vi "Adapt Cluster to Class.vi"() -> ()   [LabVIEW 2020]
doc: "This VI demonstrates a function of the GCraftsman JSON Serialization Toolkit.\n\nIt uses the 'Adapt to Type' function to convert a cluster to a LabVIEW Class Object. It performs best-fit match, handling out-of-order and missing or extra items. \nIt also successfully adapts nested objects or hierarchical class data. \n\nThis does not require the class to have accessor methods \n\nGCraftsman JSON Object Serialization Toolkit\nwww.GCraftsman.com\nCopyright (c) 2017, GCraftsman"
uses:
  Class2/Class2.lvclass
  library/JKI JSON Object Serialization.lvlib
  Class3/Class3.lvclass
  ExampleCluster.ctl
panel:
  in  "Cluster":T1={"someNumber"=123.0, "myClass3Array"=[{"myNum"=444.0}, {"myNum"=555.0}], "myBool"=TRUE, "anotherNumber"=999.0}
  out "myBool":bool
  out "anotherNumber":dbl format="%#_13g"
  out "someNumber":dbl format="%#_13g"
  out "myNum 2":dbl format="%#_13g"
  out "myNum":dbl format="%#_13g"
  out "myClass2":refnum<class "Class2.lvclass">
  # "This VI demonstrates a function of the GCraftsman JSON Serialization Toolkit.\n\nLook at the block diagram to see that the 'Adapt to Type' function can convert a cluster to a LabVIEW Class Object.   It performs best-fit match, handling out-of-order and missing or extra items.  \nIt also successfully adapts nested objects or hierarchical class data. \n\nThis does not require the class to have accessor methods"
  # "Object Data"
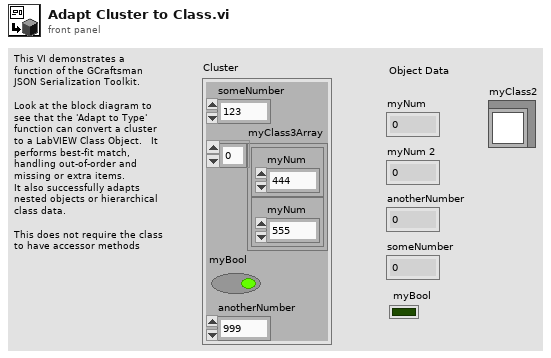
[diagram p1: front panel]
types:
  T1 = typedef "ExampleCluster.ctl" = cluster{"someNumber":dbl, "myClass3Array":cluster{"myNum":dbl}[], "myBool":bool, "anotherNumber":dbl}
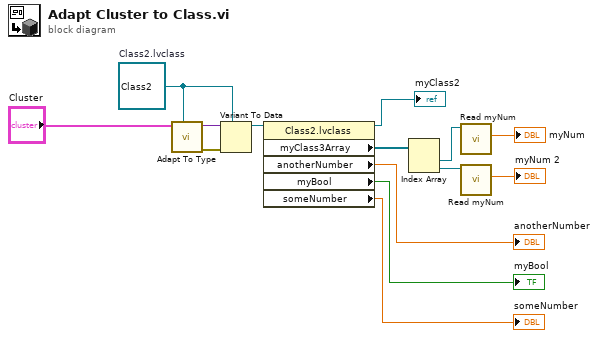
[diagram p0: block diagram]
diagram:
  w14 = refnum<class "Class2.lvclass"> refnum  # Class2.lvclass
  n1 = call "Adapt To Type.vi"("Type and Defaults"=w14, "Variant in"="Cluster") -> ("error out"=w12:errorcluster, "Variant out"=w11:variant)  [unwired: 8 in]
  n2 = Variant To Data(error in=w12, type=w14, Variant=w11) -> (data=w2:refnum<class "Class2.lvclass">)  [unwired: 1 out]
  n3 = property class="Class2.lvclass"(reference=w2) -> (reference out=→"myClass2":refnum<class "Class2.lvclass">, "myClass3Array"=w6:refnum<class "Class3.lvclass">[], "anotherNumber"=→"anotherNumber":dbl, "myBool"=→"myBool":bool, "someNumber"=→"someNumber":dbl)  [unwired: 1 in, 1 out]
  n4 = Index Array(array=w6) -> (element #1=w10:refnum<class "Class3.lvclass">, element #2=w9:refnum<class "Class3.lvclass">)  [unwired: 2 in]
  n5 = call "Read myNum.vi"("Class3 in"=w10) -> ("myNum"=→"myNum":dbl)  [unwired: 8 in, 2 out]
  n6 = call "Read myNum.vi"("Class3 in"=w9) -> ("myNum"=→"myNum 2":dbl)  [unwired: 8 in, 2 out]
